vi "Connection Close.vi"(8 "error in (no error)":errorcluster, 11 "Conection Data":T1={"VISA resource name"="COM4"}) -> (0 "error out":errorcluster, 3 "Conection Data Out":T1={"VISA resource name"="COM4"})   [LabVIEW 2014, in "SJ-210 Lib.lvlib"]
doc: "Cierra el puerto COM que indica el usuario y setea valores por defecto al puerto."
uses:
  SJ-210 Lib.lvlib
  Typedef/Connection Data.ctl
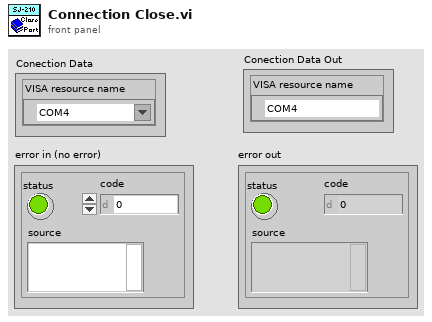
[diagram p1: front panel]
types:
  T1 = typedef "SJ-210 Lib.lvlib/Connection Data.ctl" = cluster{"VISA resource name":refnum<visa-resource-name>}
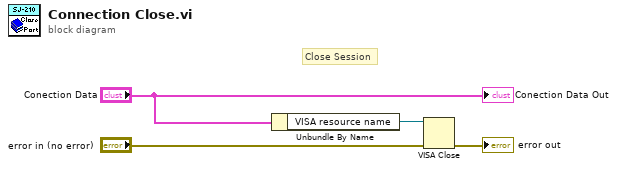
[diagram p0: block diagram]
diagram:
  # "Close Session"
  n1 = Unbundle By Name("Conection Data") -> ("VISA resource name"=w2:refnum<visa-resource-name>)
  n2 = VISA Close(VISA resource name=w2, error in (no error)="error in (no error)") -> (error out=→"error out":errorcluster)
  "Conection Data Out" <- "Conection Data"
